vi "pco.camera_Live_Example.vi"() -> ()   [LabVIEW 2020]
doc: "A short program to demonstrate the fundamentals of control and image acquision with the pco.camera series. The program records a sequence of images, with \"live\" updating, until the \"StopRecording\" button is pressed. Use ctrl-H for more help on the individual controls and indicators.\n\nCopyright 2004, 2010 The Cooke Corporation."
uses:
  <userlib>/PCO LabVIEW 5.0.0/pco.camera/Camera.lvclass
  <vilib>/picture/picture.llb/Draw 8-Bit Pixmap.vi
  <vilib>/picture/picture.llb/Draw True-Color Pixmap.vi
  <userlib>/PCO LabVIEW 5.0.0/pco.sdk/TimingControl/TimingControl.lvlib
panel:
  out "colormap(U8)":u32[](array[numeric])
  in  "Zoom [%]":i32(c297)=26
  out "Image":picture
  out "Image(U16)":u16[][](graph)
  in  "Trigger":bool
  in  "data_format":T1(ring)=enum."Mono16"
  out "rawImage":u16[][](array[numeric])
  in  "Image Index":u32 max=9
  out "Recorded Images":u32
  in  "TriggerMode":T2(ring)
  in  "Quit":bool
  out "Error":errorcluster {"code" format="%x"}
  in  "Stop Record":bool
  out "Recording On":bool
  in  "roiY1":u64=2 min=1 max=2160 step=1
  in  "roiX1":u64=2 min=1 max=2560 step=1
  in  "roiY0":u64=1 max=2159 step=1
  in  "roiX0":u64=1 max=2559 step=1
  out "Image Height":u64
  out "Image Width":u64
  in  "dwImgCount":u32=10 caption="Required Number of Images" max=2397
  in  "Exposure Time [s]":dbl=0.010000000000000002 min=0.0005 max=2.0 step=0.001
  # "This example demonstrates the image acquisition with one camera in ring buffer mode together with a live display of the latest images during record. After record is stopped, the images can be addressed by index.\nNote that this example will not be fail save, i.e. doesnt react on errors, just handles them forward to the end\n\nUsage:\nSelect your required image count, data format and the camera setup before you start the program.\nOnce started, the camera class will be initialized and images will be recorded and displayed automatically\nYou can stop the images by pressing stop record.\nAfter stopped, the image at the selected index will be read out\nTo finish the program click on quit application, this will force an exit of the camera class\nYou can change your required ROI after and also during the record."
  # "pco.labview"
  # "Camera Setup"
  # "Recording Control"
  # "Parameters for image readout"
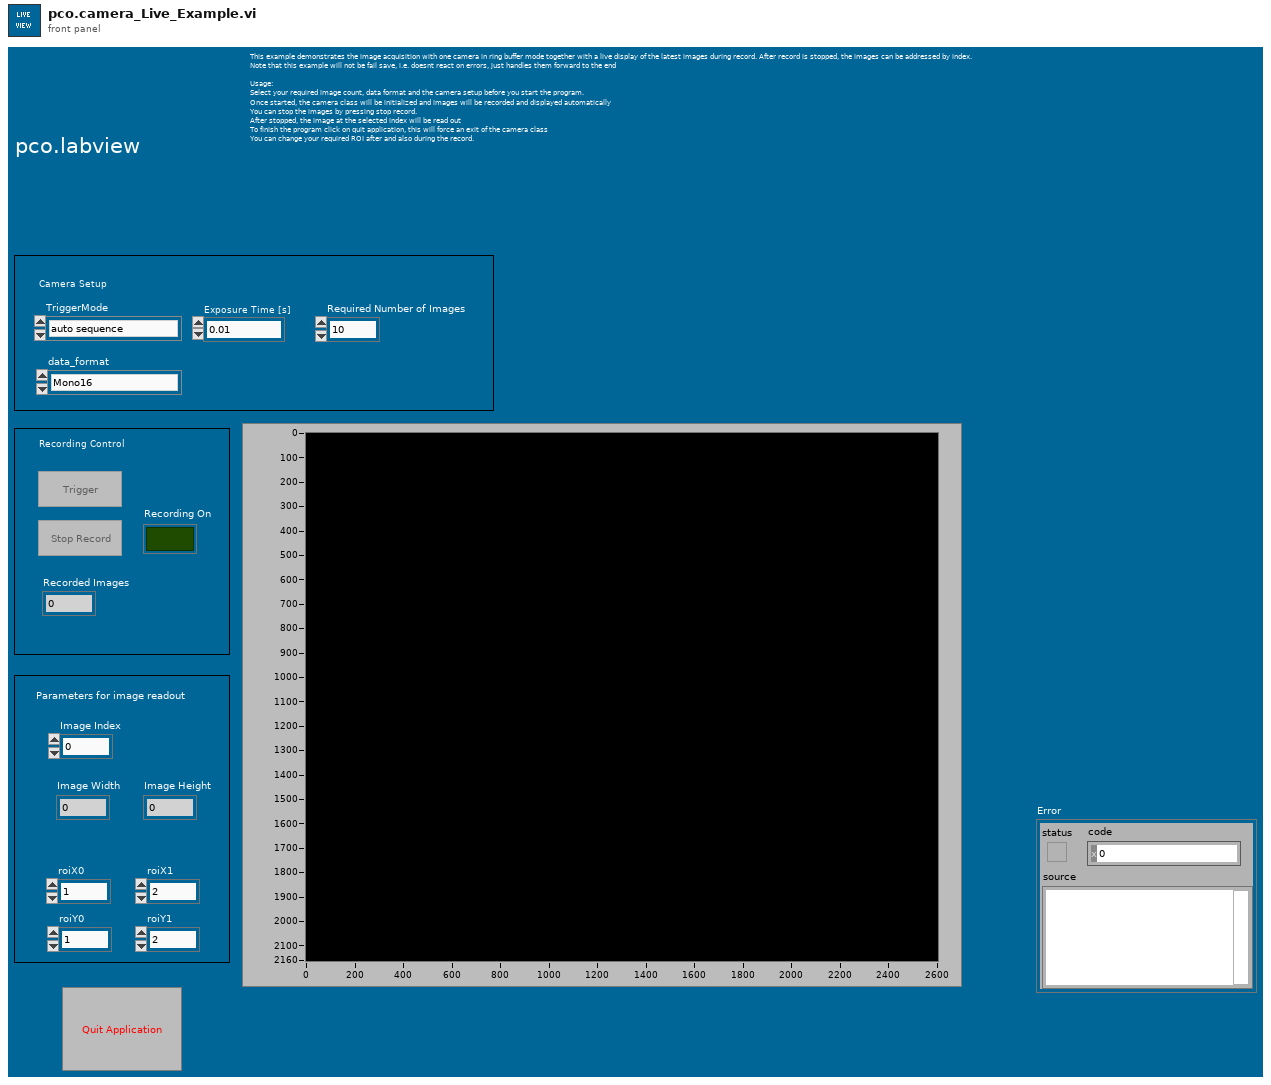
[diagram p1: front panel]
types:
  T1 = enum16{"Undefined", "Mono8", "Mono16", "BGRA8", "RGBA8", "BGRA16", "RGBA16", "CompressedMono8"}
  T2 = enum16{"auto sequence", "software trigger", "external exposure start", "external exposure control"}
  T3 = enum16{"sequence", "sequence non blocking", "ring buffer", "fifo", "sequence_dpcore", "sequence_non_blocking_dpcore", "ring_buffer_dpcore", "fifo_dpcore", "tif", "multitif", "pcoraw", "b16", "dicom", "multidicom"}
  T4 = enum8{"Enabled", "Disabled", "Disabled and Grayed Out"}
  T5 = cluster{"serial":u32, "type":u16, "sub_type":u16, "interface_type":u16, "min_exposure_time_s":dbl, "max_exposure_time_s":dbl, "min_exposure_step_s":dbl, "min_delay_time_s":dbl, "max_delay_time_s":dbl, "min_delay_step_s":dbl, "min_width":u64, "min_height":u64, "max_width":u64, "max_height":u64, "roi_step_horz":u64, "roi_step_vert":u64, "roi_symmetric_horz":bool, "roi_symmetric_vert":bool, "has_timestamp_mode":bool, "has_timestamp_mode_ascii_only":bool, "pixelrate_vec":u32[], "has_acquire_mode":bool, "has_ext_acquire_mode":bool, "has_metadata_mode":bool, "has_ram":bool, "binning_horz_vec":u16[], "binning_vert_vec":u16[]}
  T6 = typedef "Camera.lvclass/binning.ctl" = cluster{"vert":u16, "horz":u16}
  T7 = cluster{"exposure_time_s":dbl, "delay_time_s":dbl, "roi":cluster{"x0":u64, "y0":u64, "x1":u64, "y1":u64}, "timestamp_mode":u16, "pixelrate":u32, "trigger_mode":u16, "acquire_mode":u16, "metadata_mode":u16, "noisefilter_mode":u16, "binning":T6}
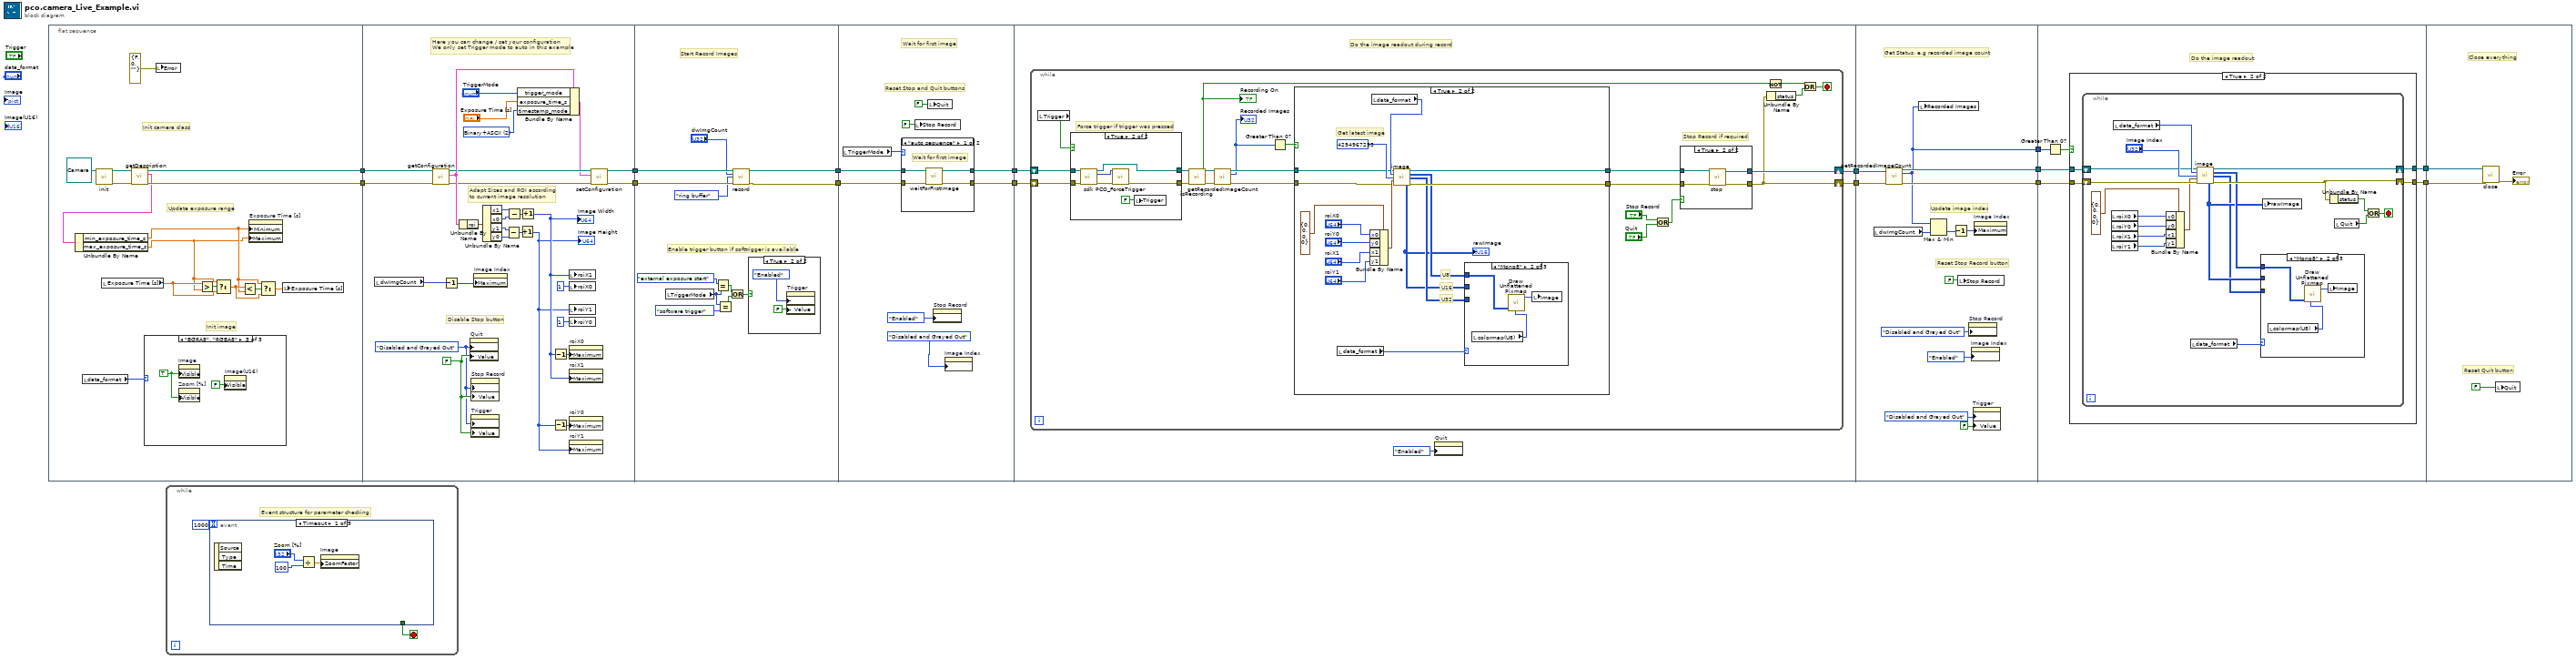
[diagram p0: block diagram]
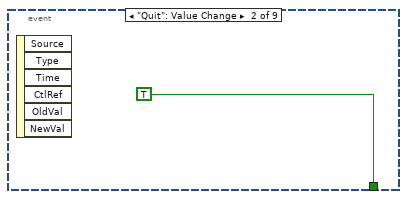
[diagram p2: hidden frame]
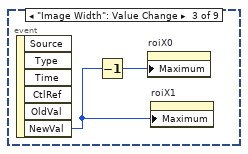
[diagram p3: hidden frame]
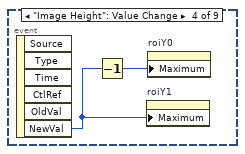
[diagram p4: hidden frame]
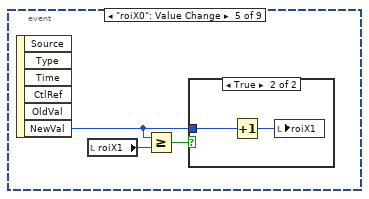
[diagram p5: hidden frame]
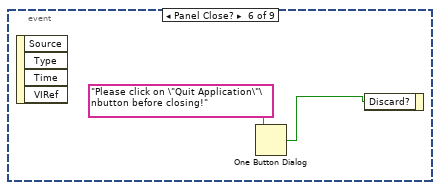
[diagram p7: hidden frame]
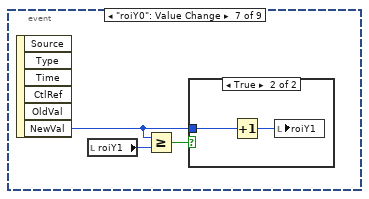
[diagram p8: hidden frame]
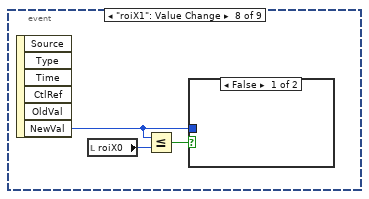
[diagram p10: hidden frame]
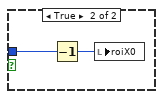
[diagram p11: hidden frame]
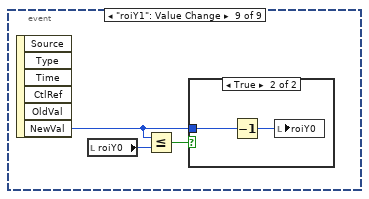
[diagram p12: hidden frame]
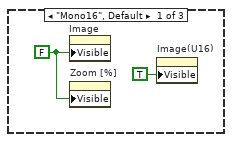
[diagram p14: hidden frame]
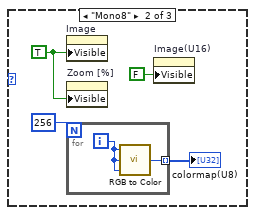
[diagram p15: hidden frame]
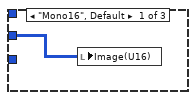
[diagram p19: hidden frame]
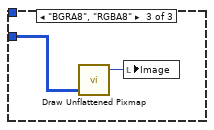
[diagram p20: hidden frame]
diagram:
  n1 = flat-sequence {
    tunnel: [w21] -> w7
    tunnel: [w20] -> w6
    tunnel: [w45] -> w15
    tunnel: [w49] -> w14
    tunnel: w7 -> [w44]
    tunnel: w6 -> [w43]
    tunnel: [w69] -> w9
    tunnel: [w70] -> w8
    tunnel: w14 -> [w80]
    tunnel: w15 -> [w79]
    tunnel: w9 -> [w87]
    tunnel: w8 -> [w88]
    tunnel: [w86] -> w13
    tunnel: [w84] -> w2
    tunnel: w13 -> [w102]
    tunnel: [w100] -> w12
    tunnel: [w99] -> w5
    tunnel: w2 -> [w98]
    tunnel: w12 -> [w173]
    tunnel: [w171] -> w11
    tunnel: w5 -> [w166]
    tunnel: [w165] -> w4
    tunnel: [w164] -> w1
    tunnel: w11 -> [w182]
    tunnel: [w181] -> w10
    tunnel: w4 -> [w180]
    tunnel: [w179] -> w3
    tunnel: w1 -> [w177]
    tunnel: w10 -> [w216]
    tunnel: w3 -> [w214]
    frame #0 {
      # "Init image"
      # "Init camera class"
      # "Update exposure range"
      n2 = local read "data_format"() -> (w16:T1)
      n3 = call-dynamic "init.vi"("Camera in"=refnum<class "Camera.lvclass"> refnum) -> ("Camera out"=w22:refnum<class "Camera.lvclass">, "error out"=w23:errorcluster)  [unwired: 8 in]
      n4 = local read "Exposure Time [s]"() -> (w29:dbl)
      n5 = call-dynamic "getDescription.vi"("error in (no error)"=w23, "Camera in"=w22) -> ("error out"=w20:errorcluster, "description"=w19:T5, "Camera out"=w21:refnum<class "Camera.lvclass">)  [unwired: 7 in]
      n6 = Unbundle By Name(w19) -> ("min_exposure_time_s"=w18:dbl, "max_exposure_time_s"=w17:dbl)
      n7 = case shown="\"BGRA8\", \"RGBA8\"" w16 {
        frame "Mono16", Default {
          w31 = FALSE ("Visible")
          n8 = property on="Image" class="Pict"("Visible"=w31) -> ()  [unwired: 2 in, 2 out]
          n9 = property on="Zoom [%]" class="Scroll (strict)"("Visible"=w31) -> ()  [unwired: 2 in, 2 out]
          n10 = property on="Image(U16)" class="IntGraph (strict)"("Visible"=TRUE) -> ()  [unwired: 2 in, 2 out]
        }
        frame "Mono8" {
          w35 = TRUE ("Visible")
          n11 = property on="Image" class="Pict"("Visible"=w35) -> ()  [unwired: 2 in, 2 out]
          n12 = property on="Zoom [%]" class="Scroll (strict)"("Visible"=w35) -> ()  [unwired: 2 in, 2 out]
          n13 = for {
            N: 256 -> [_]
            tunnel: [w37] -> w34 mode=indexing
            i -> [w38]
            n14 = call <vilib>:"RGB to Color.vi"("B"=w38, "G"=w38, "R"=w38) -> ("Color"=w37:u32)
          }
          "colormap(U8)" <- w34
          n15 = property on="Image(U16)" class="IntGraph (strict)"("Visible"=FALSE) -> ()  [unwired: 2 in, 2 out]
        }
        frame "BGRA8", "RGBA8" {
          w39 = TRUE ("Visible")
          n16 = property on="Image" class="Pict"("Visible"=w39) -> ()  [unwired: 2 in, 2 out]
          n17 = property on="Zoom [%]" class="Scroll (strict)"("Visible"=w39) -> ()  [unwired: 2 in, 2 out]
          n18 = property on="Image(U16)" class="IntGraph (strict)"("Visible"=FALSE) -> ()  [unwired: 2 in, 2 out]
        }
      }
      n19 = local write "Error"(errorcluster {"status"=FALSE, "code"=0, "source"=""} ("error IO")) -> ()
      n20 = Greater?(x=w29, y=w17) -> (0:w30:bool)
      n21 = Select(t=w17, s=w30, f=w29) -> (s? t:f=w27:dbl)
      n22 = Less?(x=w27, y=w18) -> (x < y?=w28:bool)
      n23 = property on="Exposure Time [s]" class="DigNum (strict)"("Minimum"=w18, "Maximum"=w17) -> ()  [unwired: 2 in, 2 out]
      n24 = Select(t=w18, s=w28, f=w27) -> (s? t:f=w26:dbl)
      n25 = local write "Exposure Time [s]"(w26) -> ()
    }
    frame #1 {
      w55 = u16 2 items=["OFF", "Binary", "Binary+ASCII", "ASCII"] ("wTimeStampMode")
      w42 = FALSE ("Stop")
      w41 = T4."Disabled and Grayed Out" ("Disabled")
      # "Disable Stop button"
      # "Adapt Sizes and ROI according\nto current image resolution"
      # "Here you can change / set your configuration\nWe only set Trigger mode to auto in this example"
      n26 = local read "dwImgCount"() -> (w56:u32)
      n27 = call-dynamic "getConfiguration.vi"("error in (no error)"=w43, "Camera in"=w44) -> ("error out"=w50:errorcluster, "configuration"=w61:T7, "Camera out"=w52:refnum<class "Camera.lvclass">)  [unwired: 7 in]
      n28 = Decrement(x=w56) -> (x-1=w46:u32)
      n29 = Unbundle By Name(w61) -> ("roi"=w62:cluster{"x0":u64, "y0":u64, "x1":u64, "y1":u64})
      n30 = property on="Quit" class="Bool (strict)"("DisabledEnum"=w41, "Value"=w42) -> ()  [unwired: 2 in, 2 out]
      n31 = property on="Stop Record" class="Bool (strict)"("DisabledEnum"=w41, "Value"=w42) -> ()  [unwired: 2 in, 2 out]
      n32 = property on="Trigger" class="Bool (strict)"("DisabledEnum"=w41, "Value"=w42) -> ()  [unwired: 2 in, 2 out]
      n33 = property on="Image Index" class="DigNum (strict)"("Maximum"=w46) -> ()  [unwired: 2 in, 2 out]
      n34 = Unbundle By Name(w62) -> ("x1"=w64:u64, "x0"=w63:u64, "y1"=w66:u64, "y0"=w65:u64)
      n35 = Subtract(x=w66, y=w65) -> (x-y=w68:u64)
      n36 = Subtract(x=w64, y=w63) -> (x-y=w67:u64)
      n37 = Bundle By Name(cluster=w61, "trigger_mode"="TriggerMode", "exposure_time_s"="Exposure Time [s]", "timestamp_mode"=w55) -> (w51:T7)
      n38 = Increment(x=w68) -> (x+1=w47:u64)
      "Image Height" <- w47
      n39 = Increment(x=w67) -> (x+1=w48:u64)
      "Image Width" <- w48
      n40 = Decrement(x=w48) -> (x-1=w59:u64)
      n41 = Decrement(x=w47) -> (x-1=w60:u64)
      n42 = local write "roiX1"(w48) -> ()
      n43 = local write "roiX0"(u64 1 ("roiY0")) -> ()
      n44 = local write "roiY1"(w47) -> ()
      n45 = local write "roiY0"(u64 1 ("roiY0")) -> ()
      n46 = property on="roiX0" class="DigNum (strict)"("Maximum"=w59) -> ()  [unwired: 2 in, 2 out]
      n47 = property on="roiX1" class="DigNum (strict)"("Maximum"=w48) -> ()  [unwired: 2 in, 2 out]
      n48 = property on="roiY0" class="DigNum (strict)"("Maximum"=w60) -> ()  [unwired: 2 in, 2 out]
      n49 = property on="roiY1" class="DigNum (strict)"("Maximum"=w47) -> ()  [unwired: 2 in, 2 out]
      n50 = call-dynamic "setConfiguration.vi"("error in (no error)"=w50, "configuration"=w51, "Camera in"=w52) -> ("error out"=w49:errorcluster, "Camera out"=w45:refnum<class "Camera.lvclass">)  [unwired: 7 in]
    }
    frame #2 {
      # "Enable trigger button if softtrigger is available"
      # "Start Record Images"
      n51 = local read "TriggerMode"() -> (w76:T2)
      n52 = Equal?(x=T2."external exposure start" ("TriggerMode"), y=w76) -> (x = y?=w73:bool)
      n53 = Equal?(x=w76, y=T2."software trigger" ("TriggerMode")) -> (x = y?=w72:bool)
      n54 = Or(x=w73, y=w72) -> (x .or. y?=w74:bool)
      n55 = call-dynamic "record.vi"("Camera in"=w79, "num_images"="dwImgCount", "record_mode"=T3."ring buffer", "error in (no error)"=w80) -> ("Camera out"=w70:refnum<class "Camera.lvclass">, "error out"=w69:errorcluster)  [unwired: 10 in]
      n56 = case shown="True" w74 {
        frame False {
        }
        frame True {
          n57 = property on="Trigger" class="Bool (strict)"("DisabledEnum"=T4."Enabled" ("Disabled"), "Value"=FALSE ("Trigger")) -> ()  [unwired: 2 in, 2 out]
        }
      }
    }
    frame #3 {
      # "Wait for first image"
      # "Reset Stop and Quit buttons"
      n58 = local read "TriggerMode"() -> (w83:T2)
      n59 = case shown="\"auto sequence\"" w83 {
        tunnel: w88 -> [w95 w97]
        tunnel: w87 -> [w94 w96]
        tunnel: [w93 w96] -> w86
        tunnel: [w92 w97] -> w84
        frame "auto sequence" {
          # "Wait for first image"
          n60 = call-dynamic "waitForFirstImage.vi"("error in (no error)"=w94, "Camera in"=w95) -> ("error out"=w93:errorcluster, "Camera out"=w92:refnum<class "Camera.lvclass">)  [unwired: 8 in]
        }
        frame Default {
        }
      }
      n61 = local write "Stop Record"(FALSE ("Stop Record")) -> ()
      n62 = local write "Quit"(FALSE ("Stop")) -> ()
      n63 = property on="Stop Record" class="Bool (strict)"("DisabledEnum"=T4."Enabled" ("Disabled")) -> ()  [unwired: 2 in, 2 out]
      n64 = property on="Image Index" class="DigNum (strict)"("DisabledEnum"=T4."Disabled and Grayed Out" ("Disabled")) -> ()  [unwired: 2 in, 2 out]
    }
    frame #4 {
      # "Do the image readout during record"
      n65 = while {
        shift-right: [w105] -> w100
        shift-left: w102 -> [w109]
        shift-right: [w106] -> w99
        shift-left: w98 -> [w110]
        stop <- w121 stop-if-true
        # "Force trigger if trigger was pressed"
        # "Stop Record if required"
        n66 = local read "Trigger"() -> (w111:bool)
        n67 = case shown="True" w111 {
          tunnel: w110 -> [w150 w155]
          tunnel: w109 -> [w149 w154]
          tunnel: [w150 w153] -> w108
          tunnel: [w149 w152] -> w107
          frame False {
          }
          frame True {
            n68 = call-dynamic "sdk.vi"("Camera in"=w155, "error in (no error)"=w154) -> ("Camera out"=w153:refnum<class "Camera.lvclass">, "sdk"=w156:u64, "error out"=w157:errorcluster)  [unwired: 11 in]
            n69 = call <userlib>:"PCO_ForceTrigger.vi"("error in (no error)"=w157, "ph"=w156) -> ("error out"=w152:errorcluster)  [unwired: 6 in, 3 out]
            n70 = local write "Trigger"(FALSE ("Trigger")) -> ()
          }
        }
        n71 = call-dynamic "isRecording.vi"("Camera in"=w108, "error in (no error)"=w107) -> ("Camera out"=w116:refnum<class "Camera.lvclass">, "recording"=w119:bool, "error out"=w115:errorcluster)  [unwired: 11 in]
        "Recording On" <- w119
        n72 = call-dynamic "getRecordedImageCount.vi"("Camera in"=w116, "error in (no error)"=w115) -> ("Camera out"=w113:refnum<class "Camera.lvclass">, "recorded_image_count"=w103:u32, "error out"=w114:errorcluster)  [unwired: 11 in]
        "Recorded Images" <- w103
        n73 = Greater Than 0?(x=w103) -> (x > 0?=w104:bool)
        n74 = case shown="True" w104 {
          tunnel: [w125 w137] -> w117
          tunnel: w114 -> [w125 w134]
          tunnel: w113 -> [w126 w128]
          tunnel: [w126 w127] -> w112
          frame False {
          }
          frame True {
            # "U32"
            # "U8"
            # "U16"
            # "Get latest image"
            n75 = local read "data_format"() -> (w129:T1)
            n76 = Bundle By Name(cluster=cluster{"x0":u64, "y0":u64, "x1":u64, "y1":u64} {"x0"=0, "y0"=0, "x1"=0, "y1"=0} ("roi"), "x0"="roiX0", "y0"="roiY0", "x1"="roiX1", "y1"="roiY1") -> (w138:cluster{"x0":u64, "y0":u64, "x1":u64, "y1":u64})
            n77 = local read "data_format"() -> (w133:T1)
            n78 = call-dynamic "image.vi"("Camera in"=w128, "data_format"=w133, "image_index"=u32 4294967295 ("dwImgIdx"), "roi"=w138, "error in (no error)"=w134) -> ("Camera out"=w127:refnum<class "Camera.lvclass">, "image (U8)"=w131:u8[][], "image (U32)"=w132:u32[][], "raw_image (U16)"=w130:u16[][], "error out"=w137:errorcluster)  [unwired: 3 in, 3 out]
            "rawImage" <- w130
            n79 = case shown="\"Mono8\"" w129 {
              tunnel: w132 -> [_ _ w148]
              tunnel: w131 -> [_ w146 _]
              tunnel: w130 -> [w143 _ _]
              frame "Mono16", Default {
                n80 = local write "Image(U16)"(w143) -> ()
              }
              frame "Mono8" {
                n81 = local read "colormap(U8)"() -> (w145:u32[])
                n82 = call-poly <vilib>:"Draw Unflattened Pixmap.vi"("data"=w146, "color table"=w145) -> ("new picture"=w144:picture)  [unwired: 7 in]
                n83 = local write "Image"(w144) -> ()
              }
              frame "BGRA8", "RGBA8" {
                n84 = call-poly <vilib>:"Draw Unflattened Pixmap.vi"("data (RGB format)"=w148) -> ("new picture"=w147:picture)  [unwired: 8 in]
                n85 = local write "Image"(w147) -> ()
              }
            }
          }
        }
        n86 = Or(x="Stop Record", y="Quit") -> (x .or. y?=w122:bool)
        n87 = case shown="True" w122 {
          tunnel: w117 -> [w159 w160]
          tunnel: [w158 w162] -> w106
          tunnel: [w159 w163] -> w105
          tunnel: w112 -> [w158 w161]
          frame False {
          }
          frame True {
            n88 = call-dynamic "stop.vi"("error in (no error)"=w160, "Camera in"=w161) -> ("error out"=w163:errorcluster, "Camera out"=w162:refnum<class "Camera.lvclass">)  [unwired: 8 in]
          }
        }
        n89 = Unbundle By Name(w105) -> ("status"=w120:bool)
        n90 = Not(x=w119) -> (.not. x?=w118:bool)
        n91 = Or(x=w118, y=w120) -> (x .or. y?=w121:bool)
      }
      n92 = property on="Quit" class="Bool (strict)"("DisabledEnum"=T4."Enabled" ("Disabled")) -> ()  [unwired: 2 in, 2 out]
    }
    frame #5 {
      # "Update image index"
      # "Reset Stop Record button"
      # "Get Status, e.g recorded image count"
      n93 = local read "dwImgCount"() -> (w172:u32)
      n94 = call-dynamic "getRecordedImageCount.vi"("Camera in"=w166, "error in (no error)"=w173) -> ("Camera out"=w165:refnum<class "Camera.lvclass">, "recorded_image_count"=w164:u32, "error out"=w171:errorcluster)  [unwired: 11 in]
      n95 = local write "Recorded Images"(w164) -> ()
      n96 = Max & Min(x=w164, y=w172) -> (min(x,y)=w174:u32)  [unwired: 1 out]
      n97 = Decrement(x=w174) -> (x-1=w169:u32)
      n98 = local write "Stop Record"(FALSE ("Stop Record")) -> ()
      n99 = property on="Stop Record" class="Bool (strict)"("DisabledEnum"=T4."Disabled and Grayed Out" ("Disabled")) -> ()  [unwired: 2 in, 2 out]
      n100 = property on="Image Index" class="DigNum (strict)"("DisabledEnum"=T4."Enabled" ("Disabled")) -> ()  [unwired: 2 in, 2 out]
      n101 = property on="Trigger" class="Bool (strict)"("DisabledEnum"=T4."Disabled and Grayed Out" ("Disabled"), "Value"=FALSE ("Trigger")) -> ()  [unwired: 2 in, 2 out]
      n102 = property on="Image Index" class="DigNum (strict)"("Maximum"=w169) -> ()  [unwired: 2 in, 2 out]
    }
    frame #6 {
      # "Do the image readout"
      n103 = Greater Than 0?(x=w177) -> (x > 0?=w178:bool)
      n104 = case shown="True" w178 {
        tunnel: w182 -> [w183 w188]
        tunnel: [w183 w187] -> w181
        tunnel: w180 -> [w184 w186]
        tunnel: [w184 w185] -> w179
        frame False {
        }
        frame True {
          n105 = while {
            shift-right: [w199] -> w187
            shift-left: w188 -> [w207]
            shift-right: [w193] -> w185
            shift-left: w186 -> [w194]
            stop <- w201 stop-if-true
            n106 = local read "roiX0"() -> (w197:u64)
            n107 = local read "roiY0"() -> (w198:u64)
            n108 = local read "roiX1"() -> (w205:u64)
            n109 = local read "roiY1"() -> (w204:u64)
            n110 = local read "data_format"() -> (w195:T1)
            n111 = Bundle By Name(cluster=cluster{"x0":u64, "y0":u64, "x1":u64, "y1":u64} {"x0"=0, "y0"=0, "x1"=0, "y1"=0} ("roi"), "x0"=w197, "y0"=w198, "x1"=w205, "y1"=w204) -> (w206:cluster{"x0":u64, "y0":u64, "x1":u64, "y1":u64})
            n112 = local read "data_format"() -> (w192:T1)
            n113 = call-dynamic "image.vi"("Camera in"=w194, "data_format"=w195, "image_index"="Image Index", "roi"=w206, "error in (no error)"=w207) -> ("Camera out"=w193:refnum<class "Camera.lvclass">, "image (U8)"=w191:u8[][], "image (U32)"=w189:u32[][], "raw_image (U16)"=w190:u16[][], "error out"=w199:errorcluster)  [unwired: 3 in, 3 out]
            n114 = case shown="\"Mono8\"" w192 {
              tunnel: w189 -> [_ _ w213]
              tunnel: w191 -> [_ w211 _]
              tunnel: w190 -> [w208 _ _]
              frame "Mono16", Default {
                n115 = local write "Image(U16)"(w208) -> ()
              }
              frame "Mono8" {
                n116 = local read "colormap(U8)"() -> (w210:u32[])
                n117 = call-poly <vilib>:"Draw Unflattened Pixmap.vi"("data"=w211, "color table"=w210) -> ("new picture"=w209:picture)  [unwired: 7 in]
                n118 = local write "Image"(w209) -> ()
              }
              frame "BGRA8", "RGBA8" {
                n119 = call-poly <vilib>:"Draw Unflattened Pixmap.vi"("data (RGB format)"=w213) -> ("new picture"=w212:picture)  [unwired: 8 in]
                n120 = local write "Image"(w212) -> ()
              }
            }
            n121 = local write "rawImage"(w190) -> ()
            n122 = Unbundle By Name(w199) -> ("status"=w202:bool)
            n123 = local read "Quit"() -> (w203:bool)
            n124 = Or(x=w202, y=w203) -> (x .or. y?=w201:bool)
          }
        }
      }
    }
    frame #7 {
      # "Close everything"
      # "Reset Quit button"
      n125 = call-dynamic "close.vi"("error in (no error)"=w216, "Camera in"=w214) -> ("error out"=→"Error":errorcluster)  [unwired: 9 in]
      n126 = local write "Quit"(FALSE ("Stop Record")) -> ()
    }
  }
  n127 = while {
    stop <- w218 stop-if-true
    # "Event structure for parameter checking"
    n128 = event shown="[0] Timeout" {
      selector: _ -> [_ _ _ _ _ _ _ _ _]
      dyn-events: _ -> [_ _ _ _ _ _ _ _ _]
      timeout: 1000 -> [_ _ _ _ _ _ _ _ _]
      tunnel: [_ TRUE _ _ _ _ _ _ _] -> w218
      event Timeout {
        n129 = event-data() -> ()  [unwired: 1 in, 3 out]
        n130 = Divide(x="Zoom [%]", y=100 ("Zoom [%]")) -> (x/y=w221:dbl)
        n131 = property on="Image" class="Pict"("ZoomFactor"=w221) -> ()  [unwired: 2 in, 2 out]
      }
      event "Quit": Value Change {
        n132 = event-data() -> ()  [unwired: 1 in, 6 out]
      }
      event "Image Width": Value Change {
        n133 = event-data() -> ("NewVal"=w224:u64)  [unwired: 1 in, 5 out]
        n134 = Decrement(x=w224) -> (x-1=w225:u64)
        n135 = property on="roiX0" class="DigNum (strict)"("Maximum"=w225) -> ()  [unwired: 2 in, 2 out]
        n136 = property on="roiX1" class="DigNum (strict)"("Maximum"=w224) -> ()  [unwired: 2 in, 2 out]
      }
      event "Image Height": Value Change {
        n137 = event-data() -> ("NewVal"=w226:u64)  [unwired: 1 in, 5 out]
        n138 = Decrement(x=w226) -> (x-1=w227:u64)
        n139 = property on="roiY1" class="DigNum (strict)"("Maximum"=w226) -> ()  [unwired: 2 in, 2 out]
        n140 = property on="roiY0" class="DigNum (strict)"("Maximum"=w227) -> ()  [unwired: 2 in, 2 out]
      }
      event "roiX0": Value Change {
        n141 = event-data() -> ("NewVal"=w228:u64)  [unwired: 1 in, 5 out]
        n142 = local read "roiX1"() -> (w230:u64)
        n143 = Greater Or Equal?(x=w228, y=w230) -> (x >= y?=w229:bool)
        n144 = case shown="True" w229 {
          tunnel: w228 -> [_ w232]
          frame False {
          }
          frame True {
            n145 = Increment(x=w232) -> (x+1=w231:u64)
            n146 = local write "roiX1"(w231) -> ()
          }
        }
      }
      event Panel Close? {
        n147 = event-data() -> ()  [unwired: 1 in, 4 out]
        n148 = One Button Dialog(message="Please click on \"Quit Application\"\nbutton before closing!") -> (true=w233:bool)  [unwired: 1 in]
        n149 = event-data("Discard?"=w233) -> ()  [unwired: 1 in, 1 out]
      }
      event "roiY0": Value Change {
        n150 = event-data() -> ("NewVal"=w235:u64)  [unwired: 1 in, 5 out]
        n151 = local read "roiY1"() -> (w237:u64)
        n152 = Greater Or Equal?(x=w235, y=w237) -> (x >= y?=w236:bool)
        n153 = case shown="True" w236 {
          tunnel: w235 -> [_ w239]
          frame False {
          }
          frame True {
            n154 = Increment(x=w239) -> (x+1=w238:u64)
            n155 = local write "roiY1"(w238) -> ()
          }
        }
      }
      event "roiX1": Value Change {
        n156 = event-data() -> ("NewVal"=w240:u64)  [unwired: 1 in, 5 out]
        n157 = local read "roiX0"() -> (w242:u64)
        n158 = Less Or Equal?(x=w240, y=w242) -> (x <= y?=w241:bool)
        n159 = case shown="False" w241 {
          tunnel: w240 -> [_ w244]
          frame False {
          }
          frame True {
            n160 = Decrement(x=w244) -> (x-1=w243:u64)
            n161 = local write "roiX0"(w243) -> ()
          }
        }
      }
      event "roiY1": Value Change {
        n162 = event-data() -> ("NewVal"=w245:u64)  [unwired: 1 in, 5 out]
        n163 = local read "roiY0"() -> (w247:u64)
        n164 = Less Or Equal?(x=w245, y=w247) -> (x <= y?=w246:bool)
        n165 = case shown="True" w246 {
          tunnel: w245 -> [_ w249]
          frame False {
          }
          frame True {
            n166 = Decrement(x=w249) -> (x-1=w248:u64)
            n167 = local write "roiY0"(w248) -> ()
          }
        }
      }
    }
  }
